vi "Functional Global Variable.vi"(9 "Action":T1, 11 "Initialize to":i32) -> (3 "Result":i32)   [LabVIEW 2019]
doc: "This VI is a Functional Global Variable that will take an initial value from the user, store it in the shift register, increment it then display the result in an indicator"
uses:
  Action Items.ctl
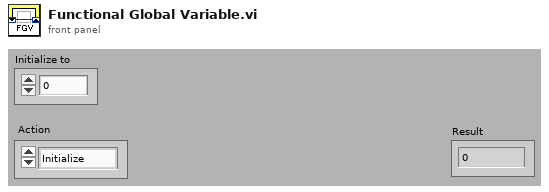
[diagram p1: front panel]
types:
  T1 = typedef "Action Items.ctl" = enum16{"Initialize", "Get", "Increment"}
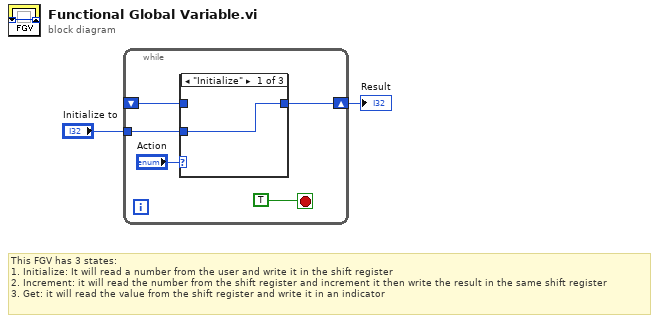
[diagram p0: block diagram]
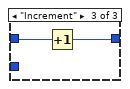
[diagram p3: hidden frame]
diagram:
  # "This FGV has 3 states:\n1. Initialize: It will read a number from the user and write it in the shift register\n2. Increment: it will read the number from the shift register and increment it then write the result in the same shift register\n3. Get: it will read the value from the shift register and write it in an indicator"
  n1 = while {
    shift-right: [w7] -> w1
    shift-left: _ -> [w6]
    tunnel: "Initialize to" -> [w3]
    stop <- TRUE ("stop") stop-if-true
    n2 = case shown="\"Initialize\"" "Action" {
      tunnel: [w8 w9 w10] -> w7
      tunnel: w6 -> [_ w9 w11]
      tunnel: w3 -> [w8 _ _]
      frame "Initialize" {
      }
      frame "Get" {
      }
      frame "Increment" {
        n3 = Increment(x=w11) -> (x+1=w10:i32)
      }
    }
  }
  "Result" <- w1
